vi "DestroySyncRefnums.vi"(8 "error in (no error)":errorcluster, 11 "ModuleAdmin":refnum<class "ModuleAdmin.lvclass">) -> (0 "error out":errorcluster)   [LabVIEW 2018, in "ModuleAdmin.lvlib" / "ModuleAdmin.lvclass"]
uses:
  ModuleAdmin.lvclass
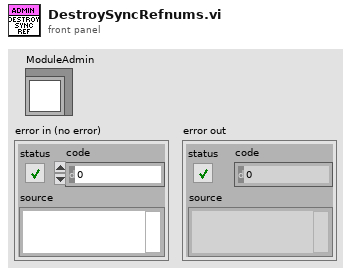
[diagram p1: front panel]
types:
  T1 = typedef "Rendezvous RefNum" = refnum<k1>
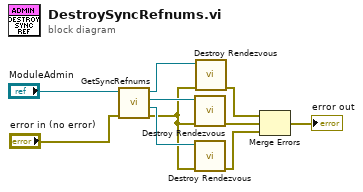
[diagram p0: block diagram]
diagram:
  n1 = call "GetSyncRefnums.vi"("error in (no error)"="error in (no error)", "ModuleAdmin"="ModuleAdmin") -> ("error out"=w6:errorcluster, "rndzv_ModuleSync"=w7:T1, "rndzv_EventSync"=w8:T1, "rndzv_StopSync"=w9:T1)  [unwired: 6 in]
  n2 = call <vilib>:"Destroy Rendezvous.vi"("error in (no error)"=w6, "rendezvous"=w8) -> ("error out"=w5:errorcluster)  [unwired: 4 in, 1 out]
  n3 = call <vilib>:"Destroy Rendezvous.vi"("error in (no error)"=w6, "rendezvous"=w7) -> ("error out"=w4:errorcluster)  [unwired: 4 in, 1 out]
  n4 = call <vilib>:"Destroy Rendezvous.vi"("error in (no error)"=w6, "rendezvous"=w9) -> ("error out"=w3:errorcluster)  [unwired: 4 in, 1 out]
  n5 = Merge Errors(w3, w5, w4) -> (→"error out":errorcluster)
